vi "DilutionWalker.vi"() -> ()   [LabVIEW 2021]
uses:
  <userlib>/Nanonis Prog Interface V5/Nanonis Prog Interface.lvlib
panel:
  in  "Lockin offset (V)":dbl
  out "End":bool
  out "Pause":bool
  out "STM RX Temp":dbl=4.40353
  in  "STM RX\nTemperature Limit (K)":dbl=5.0
  out "Mix Chamber Temp":dbl=0.372436
  in  "Wait time (ms)":i32=1000
  in  "X Cap Upper limit (mV)":dbl=0.285
  in  "X Cap Lower limit (mV)":dbl=0.21
  in  "Mixing Chamber\nTemperature Limit (K)":dbl=0.4
  in  "?":bool
  in  "Number of Steps Increment":i32=400
  out "Z capacitance (pA)":cluster{"y":i32, sgl}[](graph)=[{"y"=0, -0.26452944}, {"y"=200, -0.27056125}, {"y"=400, -0.3170625}, {"y"=600, -0.30098757}, {"y"=800, -0.3354134}, {"y"=1000, -0.29213223}, {"y"=1200, -0.30642745}, {"y"=1400, -0.29814354}, {"y"=1600, -0.30608574}, {"y"=1800, -0.25005463}, {"y"=2000, -0.24961738}, {"y"=2200, -0.3531282}, {"y"=2400, -0.30892673}, {"y"=2600, -0.33144677}, {"y"=2800, -0.3248681}, {"y"=3000, -0.3031656}, {"y"=3200, -0.30311397}, {"y"=3400, -0.3312512}, {"y"=3600, -0.31709746}, {"y"=3800, -0.25381535}, {"y"=4000, -0.29973197}, {"y"=4200, -0.25194013}, {"y"=4400, -0.27562597}, {"y"=4600, -0.27429092}, {"y"=4800, -0.32395697}, {"y"=5000, -0.23664412}, {"y"=5200, -0.2965325}, {"y"=5400, -0.22288579}, {"y"=5600, -0.28061736}, {"y"=5800, -0.27647328}, {"y"=6000, -0.32065016}, {"y"=6200, -0.31318536}, {"y"=6400, -0.32285127}, {"y"=6600, -0.31599003}, {"y"=6800, -0.30435067}, {"y"=7000, -0.31278306}, {"y"=7200, -0.3015731}, {"y"=7400, -0.23340864}, {"y"=7600, -0.31077635}, {"y"=7800, -0.30132312}, {"y"=8000, -0.27798784}, {"y"=8200, -0.33925742}, {"y"=8400, -0.28044957}, {"y"=8600, -0.27736}, {"y"=8800, -0.26748103}, {"y"=9000, -0.26297227}, {"y"=9200, -0.35384896}, {"y"=9400, -0.28351077}, {"y"=9600, -0.27015728}, {"y"=9800, -0.2900495}, {"y"=10000, -0.30096906}, {"y"=10200, -0.34584683}, {"y"=10400, -0.33333805}, {"y"=10600, -0.25753516}, {"y"=10800, -0.32054728}, {"y"=11000, -0.33541495}, {"y"=11200, -0.30325446}, {"y"=11400, -0.24681602}, {"y"=11600, -0.28720984}, {"y"=11800, -0.32199413}, {"y"=12000, -0.34654015}, {"y"=12200, -0.25113922}, {"y"=12400, -0.31027225}, {"y"=12600, -0.2965383}, {"y"=12800, -0.314928}, {"y"=13000, -0.34754327}, {"y"=13200, -0.2174063}, {"y"=13400, -0.3269226}, {"y"=13600, -0.3417576}, {"y"=13800, -0.34317303}, {"y"=14000, -0.30799103}, {"y"=14200, -0.3409932}, {"y"=14400, -0.374583}, {"y"=14600, -0.3127186}, {"y"=14800, -0.36349568}, {"y"=15000, -0.32258537}, {"y"=15200, -0.35234475}, {"y"=15400, -0.26450554}, {"y"=15600, -0.31535837}, {"y"=15800, -0.29797876}, {"y"=16000, -0.37099135}, {"y"=16200, -0.3595007}, {"y"=16400, -0.3029738}, {"y"=16600, -0.3430387}, {"y"=16800, -0.32379654}, {"y"=17000, -0.2897029}, {"y"=17200, -0.35686213}, {"y"=17400, -0.32995725}, {"y"=17600, -0.3243773}, {"y"=17800, -0.27956468}, {"y"=18000, -0.33224046}, {"y"=18200, -0.26174507}, {"y"=18400, -0.2720899}, {"y"=18600, -0.31190276}, {"y"=18800, -0.365169}, {"y"=19000, -0.35901952}, {"y"=19200, -0.3133453}, {"y"=19400, -0.321272}, {"y"=19600, -0.3650524}, {"y"=19800, -0.3569558}, {"y"=20000, -0.3226467}, {"y"=20200, -0.3186869}, {"y"=20400, -0.27690017}, {"y"=20600, -0.29333174}, {"y"=20800, -0.3650037}, {"y"=21000, -0.34175736}, {"y"=21200, -0.30235806}, {"y"=21400, -0.30519643}, {"y"=21600, -0.33016568}, {"y"=21800, -0.268843}, {"y"=22000, -0.30949652}, {"y"=22200, -0.3402042}, {"y"=22400, -0.31630984}, {"y"=22600, -0.35675278}, {"y"=22800, -0.38607332}, {"y"=23000, -0.30069488}, {"y"=23200, -0.30392653}, {"y"=23400, -0.30562043}, {"y"=23600, -0.32636446}, {"y"=23800, -0.35105774}, {"y"=24000, -0.352251}, {"y"=24200, -0.27246413}, {"y"=24400, -0.32045224}, {"y"=24600, -0.30963522}, {"y"=24800, -0.3008064}, {"y"=25000, -0.2882819}, {"y"=25200, -0.24162695}, {"y"=25400, -0.3588808}, {"y"=25600, -0.37624997}, {"y"=25800, -0.33530983}, {"y"=26000, -0.32908398}, {"y"=26200, -0.36574924}, {"y"=26400, -0.36143667}, {"y"=26600, -0.31042248}, {"y"=26800, -0.28622916}, {"y"=27000, -0.32861832}, {"y"=27200, -0.35194245}, {"y"=27400, -0.2839697}, {"y"=27600, -0.3729146}, {"y"=27800, -0.35619572}, {"y"=28000, -0.31095412}, {"y"=28200, -0.32930008}, {"y"=28400, -0.3850868}, {"y"=28600, -0.3546264}, {"y"=28800, -0.29183277}, {"y"=29000, -0.25951427}, {"y"=29200, -0.34055057}, {"y"=29400, -0.30871165}, {"y"=29600, -0.33900478}, {"y"=29800, -0.26332897}, {"y"=30000, -0.34367266}, {"y"=30200, -0.3274469}, {"y"=30400, -0.3054115}, {"y"=30600, -0.27346995}, {"y"=30800, -0.3273148}, {"y"=31000, -0.30582932}, {"y"=31200, -0.27342635}, {"y"=31400, -0.3353544}, {"y"=31600, -0.3352716}, {"y"=31800, -0.31236312}, {"y"=32000, -0.29076076}, {"y"=32200, -0.30152094}, {"y"=32400, -0.35034788}, {"y"=32600, -0.265896}, {"y"=32800, -0.31590983}, {"y"=33000, -0.31764394}, {"y"=33200, -0.3159363}, {"y"=33400, -0.34009102}, {"y"=33600, -0.29582712}, {"y"=33800, -0.3217109}, {"y"=34000, -0.25372702}, {"y"=34200, -0.24392112}, {"y"=34400, -0.28812993}, {"y"=34600, -0.28951606}, {"y"=34800, -0.3079025}, {"y"=35000, -0.33620673}, {"y"=35200, -0.292474}, {"y"=35400, -0.3607892}, {"y"=35600, -0.27421385}, {"y"=35800, -0.3280191}, {"y"=36000, -0.302316}, {"y"=36200, -0.32416925}, {"y"=36400, -0.34789872}, {"y"=36600, -0.3196872}, {"y"=36800, -0.32483512}, {"y"=37000, -0.26164752}, {"y"=37200, -0.2820668}, {"y"=37400, -0.30672884}, {"y"=37600, -0.3690237}, {"y"=37800, -0.30537617}, {"y"=38000, -0.3308374}, {"y"=38200, -0.31725284}, {"y"=38400, -0.36457232}, {"y"=38600, -0.3042373}, {"y"=38800, -0.30165693}, {"y"=39000, -0.33604917}, {"y"=39200, -0.35489634}, {"y"=39400, -0.2743292}, {"y"=39600, -0.29021338}, {"y"=39800, -0.30953702}, {"y"=40000, -0.3207827}, {"y"=40200, -0.3375588}, {"y"=40400, -0.21972783}, {"y"=40600, -0.33964434}, {"y"=40800, -0.27738118}, {"y"=41000, -0.29640958}, {"y"=41200, -0.3743232}, {"y"=41400, -0.25270778}, {"y"=41600, -0.3212443}, {"y"=41800, -0.2828819}, {"y"=42000, -0.32858887}, {"y"=42200, -0.31920588}, {"y"=42400, -0.28080276}, {"y"=42600, -0.3156575}, {"y"=42800, -0.29654214}, {"y"=43000, -0.334953}, {"y"=43200, -0.33291087}, {"y"=43400, -0.33731157}, {"y"=43600, -0.29409498}, {"y"=43800, -0.29746836}, {"y"=44000, -0.31584385}, {"y"=44200, -0.39908078}, {"y"=44400, -0.28772417}, {"y"=44600, -0.28497294}, {"y"=44800, -0.28721952}, {"y"=45000, -0.31769314}, {"y"=45200, -0.25906157}, {"y"=45400, -0.3401025}, {"y"=45600, -0.2770137}, {"y"=45800, -0.30092195}, {"y"=46000, -0.30380133}, {"y"=46200, -0.33371064}, {"y"=46400, -0.3082187}, {"y"=46600, -0.36706933}, {"y"=46800, -0.28566322}, {"y"=47000, -0.30453646}, {"y"=47200, -0.2129875}, {"y"=47400, -0.35215983}, {"y"=47600, -0.30520058}, {"y"=47800, -0.38486058}, {"y"=48000, -0.30373412}, {"y"=48200, -0.3050348}, {"y"=48400, -0.25940648}, {"y"=48600, -0.3414501}, {"y"=48800, -0.29289445}, {"y"=49000, -0.3197257}, {"y"=49200, -0.28932348}, {"y"=49400, -0.26191166}, {"y"=49600, -0.19608292}, {"y"=49800, -0.3571897}, {"y"=50000, -0.32131934}, {"y"=50200, -0.30441958}, {"y"=50400, -0.32406878}, {"y"=50600, -0.34500462}, {"y"=50800, -0.34577286}, {"y"=51000, -0.27084503}, {"y"=51200, 0.008703331}, {"y"=51400, -0.5370679}, {"y"=51600, -0.28328782}, {"y"=51800, -0.31837463}, {"y"=52000, -0.28617984}, {"y"=52200, -0.2819138}, {"y"=52400, -0.31492892}, {"y"=52600, -0.28859508}, {"y"=52800, -0.30150834}, {"y"=53000, -0.26601008}, {"y"=53200, -0.28601724}, {"y"=53400, -0.2551962}, {"y"=53600, -0.30998704}, {"y"=53800, -0.29331136}, {"y"=54000, -0.24365473}, {"y"=54200, -0.2894879}]
  out "X capacitance (mV)":cluster{"y":i32, dbl}[](graph)=[{"y"=0, 0.21357266902923586}, {"y"=200, 0.2147012710571289}, {"y"=400, 0.21581780910491943}, {"y"=600, 0.21690545082092286}, {"y"=800, 0.2179858684539795}, {"y"=1000, 0.21903662681579592}, {"y"=1200, 0.22008056640625}, {"y"=1400, 0.22109785079956054}, {"y"=1600, 0.22207918167114257}, {"y"=1800, 0.2231245517730713}, {"y"=2000, 0.2240769386291504}, {"y"=2200, 0.22501637935638427}, {"y"=2400, 0.22596323490142822}, {"y"=2600, 0.2268744945526123}, {"y"=2800, 0.22776687145233154}, {"y"=3000, 0.22866487503051758}, {"y"=3200, 0.229524302482605}, {"y"=3400, 0.23036799430847169}, {"y"=3600, 0.2312250852584839}, {"y"=3800, 0.23205804824829102}, {"y"=4000, 0.23286981582641603}, {"y"=4200, 0.23366889953613282}, {"y"=4400, 0.234482216835022}, {"y"=4600, 0.23526401519775392}, {"y"=4800, 0.23600375652313232}, {"y"=5000, 0.23675258159637452}, {"y"=5200, 0.23748691082000734}, {"y"=5400, 0.2381901264190674}, {"y"=5600, 0.2389019250869751}, {"y"=5800, 0.23960814476013184}, {"y"=6000, 0.24029965400695802}, {"y"=6200, 0.24096741676330566}, {"y"=6400, 0.24164459705352784}, {"y"=6600, 0.2423039197921753}, {"y"=6800, 0.24296264648437502}, {"y"=7000, 0.24360923767089845}, {"y"=7200, 0.2442251205444336}, {"y"=7400, 0.24485447406768798}, {"y"=7600, 0.2454981565475464}, {"y"=7800, 0.24609751701354982}, {"y"=8000, 0.2466892719268799}, {"y"=8200, 0.24729080200195314}, {"y"=8400, 0.2478795051574707}, {"y"=8600, 0.24845747947692873}, {"y"=8800, 0.24902808666229248}, {"y"=9000, 0.24959423542022705}, {"y"=9200, 0.2501417398452759}, {"y"=9400, 0.2507206678390503}, {"y"=9600, 0.25126259326934813}, {"y"=9800, 0.25181381702423095}, {"y"=10000, 0.2523436784744263}, {"y"=10200, 0.25286843776702883}, {"y"=10400, 0.2534111738204956}, {"y"=10600, 0.25392258167266846}, {"y"=10800, 0.2544567346572876}, {"y"=11000, 0.254944896697998}, {"y"=11200, 0.2554523706436157}, {"y"=11400, 0.2559502363204956}, {"y"=11600, 0.2564888000488281}, {"y"=11800, 0.2569794416427612}, {"y"=12000, 0.2574486017227173}, {"y"=12200, 0.25792760848999025}, {"y"=12400, 0.2583930253982544}, {"y"=12600, 0.2588639259338379}, {"y"=12800, 0.25932180881500244}, {"y"=13000, 0.25977411270141604}, {"y"=13200, 0.26023385524749754}, {"y"=13400, 0.2606536626815796}, {"y"=13600, 0.26108036041259763}, {"y"=13800, 0.2615255832672119}, {"y"=14000, 0.26193556785583494}, {"y"=14200, 0.2623560428619385}, {"y"=14400, 0.26276822090148927}, {"y"=14600, 0.2631711483001709}, {"y"=14800, 0.2635857343673706}, {"y"=15000, 0.26398282051086425}, {"y"=15200, 0.26438772678375244}, {"y"=15400, 0.26477880477905275}, {"y"=15600, 0.2651677131652832}, {"y"=15800, 0.26553940773010254}, {"y"=16000, 0.2659076929092407}, {"y"=16200, 0.2662929058074951}, {"y"=16400, 0.26666946411132814}, {"y"=16600, 0.2670249938964844}, {"y"=16800, 0.2674261569976807}, {"y"=17000, 0.2678008794784546}, {"y"=17200, 0.26815156936645507}, {"y"=17400, 0.26851491928100585}, {"y"=17600, 0.26885788440704345}, {"y"=17800, 0.2691839694976807}, {"y"=18000, 0.26951904296875}, {"y"=18200, 0.2698603868484497}, {"y"=18400, 0.27021329402923583}, {"y"=18600, 0.2705530643463135}, {"y"=18800, 0.2708828210830689}, {"y"=19000, 0.2712192296981812}, {"y"=19200, 0.2715223789215088}, {"y"=19400, 0.2718502998352051}, {"y"=19600, 0.2721735954284668}, {"y"=19800, 0.2724856615066528}, {"y"=20000, 0.27282190322875977}, {"y"=20200, 0.2731217622756958}, {"y"=20400, 0.27344110012054446}, {"y"=20600, 0.27374932765960697}, {"y"=20800, 0.27404532432556156}, {"y"=21000, 0.27433764934539795}, {"y"=21200, 0.2746425151824951}, {"y"=21400, 0.2749338150024414}, {"y"=21600, 0.2752199411392212}, {"y"=21800, 0.27551238536834716}, {"y"=22000, 0.2758016586303711}, {"y"=22200, 0.2760864019393921}, {"y"=22400, 0.27636544704437255}, {"y"=22600, 0.27662317752838134}, {"y"=22800, 0.2768929719924927}, {"y"=23000, 0.2771783828735352}, {"y"=23200, 0.2774518013000488}, {"y"=23400, 0.27770495414733887}, {"y"=23600, 0.27798678874969485}, {"y"=23800, 0.27826545238494876}, {"y"=24000, 0.27853381633758545}, {"y"=24200, 0.27880263328552246}, {"y"=24400, 0.27903494834899906}, {"y"=24600, 0.2792867183685303}, {"y"=24800, 0.27953026294708255}, {"y"=25000, 0.27976553440093993}, {"y"=25200, 0.27997915744781493}, {"y"=25400, 0.2802250385284424}, {"y"=25600, 0.2804482221603394}, {"y"=25800, 0.28068132400512696}, {"y"=26000, 0.28090481758117675}, {"y"=26200, 0.2811241865158081}, {"y"=26400, 0.28135080337524415}, {"y"=26600, 0.28156116008758547}, {"y"=26800, 0.2817727088928223}, {"y"=27000, 0.28198957443237305}, {"y"=27200, 0.2822116374969483}, {"y"=27400, 0.28240485191345216}, {"y"=27600, 0.28261585235595704}, {"y"=27800, 0.2828121900558472}, {"y"=28000, 0.28301324844360354}, {"y"=28200, 0.2831972360610962}, {"y"=28400, 0.28341150283813477}, {"y"=28600, 0.2835517644882202}, {"y"=28800, 0.28375835418701173}, {"y"=29000, 0.28395938873291016}, {"y"=29200, 0.2841550588607788}, {"y"=29400, 0.28433682918548586}, {"y"=29600, 0.284511923789978}, {"y"=29800, 0.28469271659851075}, {"y"=30000, 0.2848948955535889}, {"y"=30200, 0.28506882190704347}, {"y"=30400, 0.2852374076843262}, {"y"=30600, 0.2854273080825806}, {"y"=30800, 0.2855900764465332}, {"y"=31000, 0.28576691150665284}, {"y"=31200, 0.2859371662139893}, {"y"=31400, 0.2861051082611084}, {"y"=31600, 0.2862806081771851}, {"y"=31800, 0.2864513874053955}, {"y"=32000, 0.28663358688354496}, {"y"=32200, 0.2867846727371216}, {"y"=32400, 0.2869489431381226}, {"y"=32600, 0.2871151685714722}, {"y"=32800, 0.2872730016708374}, {"y"=33000, 0.28744561672210694}, {"y"=33200, 0.2875957250595093}, {"y"=33400, 0.2877490758895874}, {"y"=33600, 0.28789725303649905}, {"y"=33800, 0.2880505323410034}, {"y"=34000, 0.2882134437561035}, {"y"=34200, 0.2883355140686035}, {"y"=34400, 0.2884969234466553}, {"y"=34600, 0.28863437175750734}, {"y"=34800, 0.28878488540649416}, {"y"=35000, 0.2889194250106812}, {"y"=35200, 0.2890756130218506}, {"y"=35400, 0.2892141819000244}, {"y"=35600, 0.2894058465957642}, {"y"=35800, 0.28953988552093507}, {"y"=36000, 0.28968157768249514}, {"y"=36200, 0.2898248672485352}, {"y"=36400, 0.28995480537414553}, {"y"=36600, 0.2900970697402954}, {"y"=36800, 0.29024991989135746}, {"y"=37000, 0.2903444528579712}, {"y"=37200, 0.29047365188598634}, {"y"=37400, 0.2906097650527954}, {"y"=37600, 0.29073963165283206}, {"y"=37800, 0.29086334705352784}, {"y"=38000, 0.29100320339202884}, {"y"=38200, 0.2911355495452881}, {"y"=38400, 0.2912521123886109}, {"y"=38600, 0.29138960838317873}, {"y"=38800, 0.29152185916900636}, {"y"=39000, 0.29163422584533694}, {"y"=39200, 0.2917720556259155}, {"y"=39400, 0.2919000625610352}, {"y"=39600, 0.29201946258544925}, {"y"=39800, 0.2921566724777222}, {"y"=40000, 0.29228351116180423}, {"y"=40200, 0.2924021005630493}, {"y"=40400, 0.29252257347106936}, {"y"=40600, 0.29265565872192384}, {"y"=40800, 0.2927766084671021}, {"y"=41000, 0.2928893804550171}, {"y"=41200, 0.29299316406250003}, {"y"=41400, 0.293117880821228}, {"y"=41600, 0.29324495792388916}, {"y"=41800, 0.29335086345672606}, {"y"=42000, 0.2934612512588501}, {"y"=42200, 0.2935697317123413}, {"y"=42400, 0.29368646144866944}, {"y"=42600, 0.29380550384521487}, {"y"=42800, 0.293912148475647}, {"y"=43000, 0.2940265417098999}, {"y"=43200, 0.2941251277923584}, {"y"=43400, 0.2942491054534912}, {"y"=43600, 0.29435300827026367}, {"y"=43800, 0.29446349143981937}, {"y"=44000, 0.29457106590271}, {"y"=44200, 0.2946788311004639}, {"y"=44400, 0.2947965145111084}, {"y"=44600, 0.2949222087860108}, {"y"=44800, 0.29503176212310794}, {"y"=45000, 0.2951323747634888}, {"y"=45200, 0.29524805545806887}, {"y"=45400, 0.2953538417816162}, {"y"=45600, 0.29539966583251953}, {"y"=45800, 0.2955051898956299}, {"y"=46000, 0.29560346603393556}, {"y"=46200, 0.2957145929336548}, {"y"=46400, 0.29580819606781006}, {"y"=46600, 0.29591619968414307}, {"y"=46800, 0.2960115909576416}, {"y"=47000, 0.29612088203430176}, {"y"=47200, 0.2962247610092163}, {"y"=47400, 0.29632201194763186}, {"y"=47600, 0.2964148044586182}, {"y"=47800, 0.296518611907959}, {"y"=48000, 0.29661657810211184}, {"y"=48200, 0.2967301368713379}, {"y"=48400, 0.29681997299194335}, {"y"=48600, 0.29692456722259525}, {"y"=48800, 0.2970076322555542}, {"y"=49000, 0.2971181392669678}, {"y"=49200, 0.29723029136657714}, {"y"=49400, 0.2972947359085083}, {"y"=49600, 0.2974052667617798}, {"y"=49800, 0.29750559329986576}, {"y"=50000, 0.2976086616516113}, {"y"=50200, 0.29770348072052005}, {"y"=50400, 0.2977898597717285}, {"y"=50600, 0.297877836227417}, {"y"=50800, 0.297983193397522}, {"y"=51000, 0.29804625511169436}, {"y"=51200, 0.29815452098846434}, {"y"=51400, 0.29822735786437987}, {"y"=51600, 0.2983759164810181}, {"y"=51800, 0.29846811294555664}, {"y"=52000, 0.2985581159591675}, {"y"=52200, 0.2986560583114624}, {"y"=52400, 0.2987450838088989}, {"y"=52600, 0.298833703994751}, {"y"=52800, 0.29891486167907716}, {"y"=53000, 0.2989931344985962}, {"y"=53200, 0.2990796804428101}, {"y"=53400, 0.29915268421173097}, {"y"=53600, 0.2992403984069824}, {"y"=53800, 0.29933180809021}, {"y"=54000, 0.29941155910491946}, {"y"=54200, 0.2994891405105591}]
  in  "Lockin sensitivity (V)":dbl=0.001
  out "X capacitance (mV)":sgl=0.29948914
  out "Current (pA)":sgl=0.15895681
  out "Z capacitance (pA)":sgl=-0.2894879
  # "+X"
  # "-X"
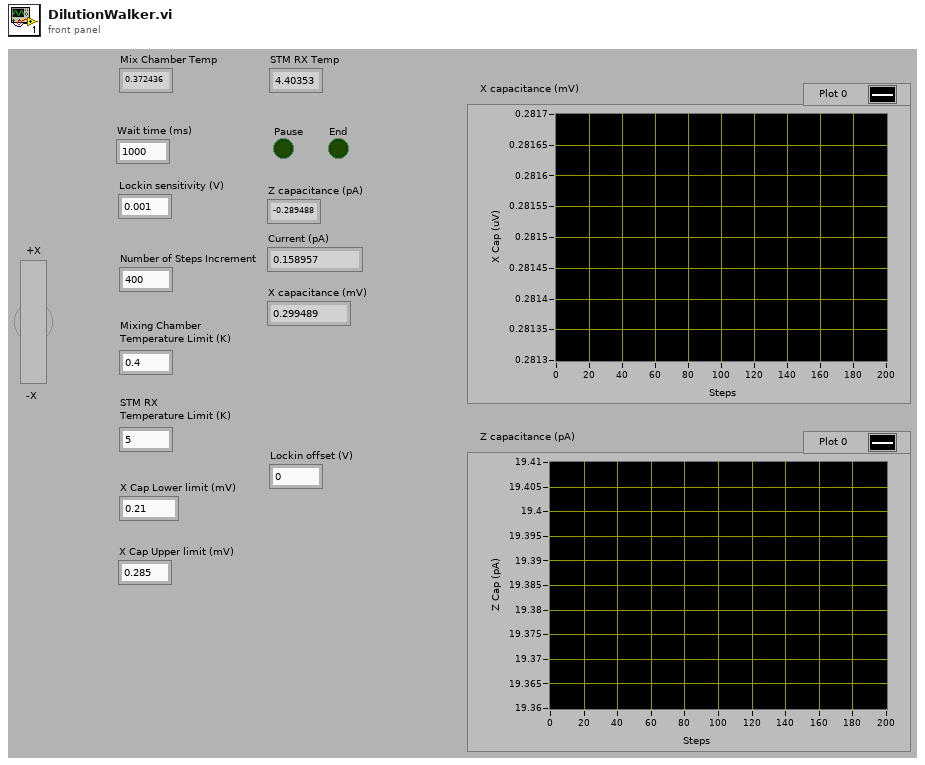
[diagram p1: front panel]
types:
  T1 = enum16{"Set Heater Voltage", "Read Heater Voltage", "Read Heater Current", "Read 1K Pot Temperature", "Read IVC Sorb Temperature", "Read Needle Valve Temperature", "Read Still Pressure", "Read Mixing Chamber Temperature", "Read STM RX Temperature", "Read STM CX Temperature", "Unstall Triton Loop", "Triton Stop", "Triton Stall Status"}
  T2 = enum8{"Group 1", "Group 2", "Group 3", "Group 4", "Group 5", "Group 6"}
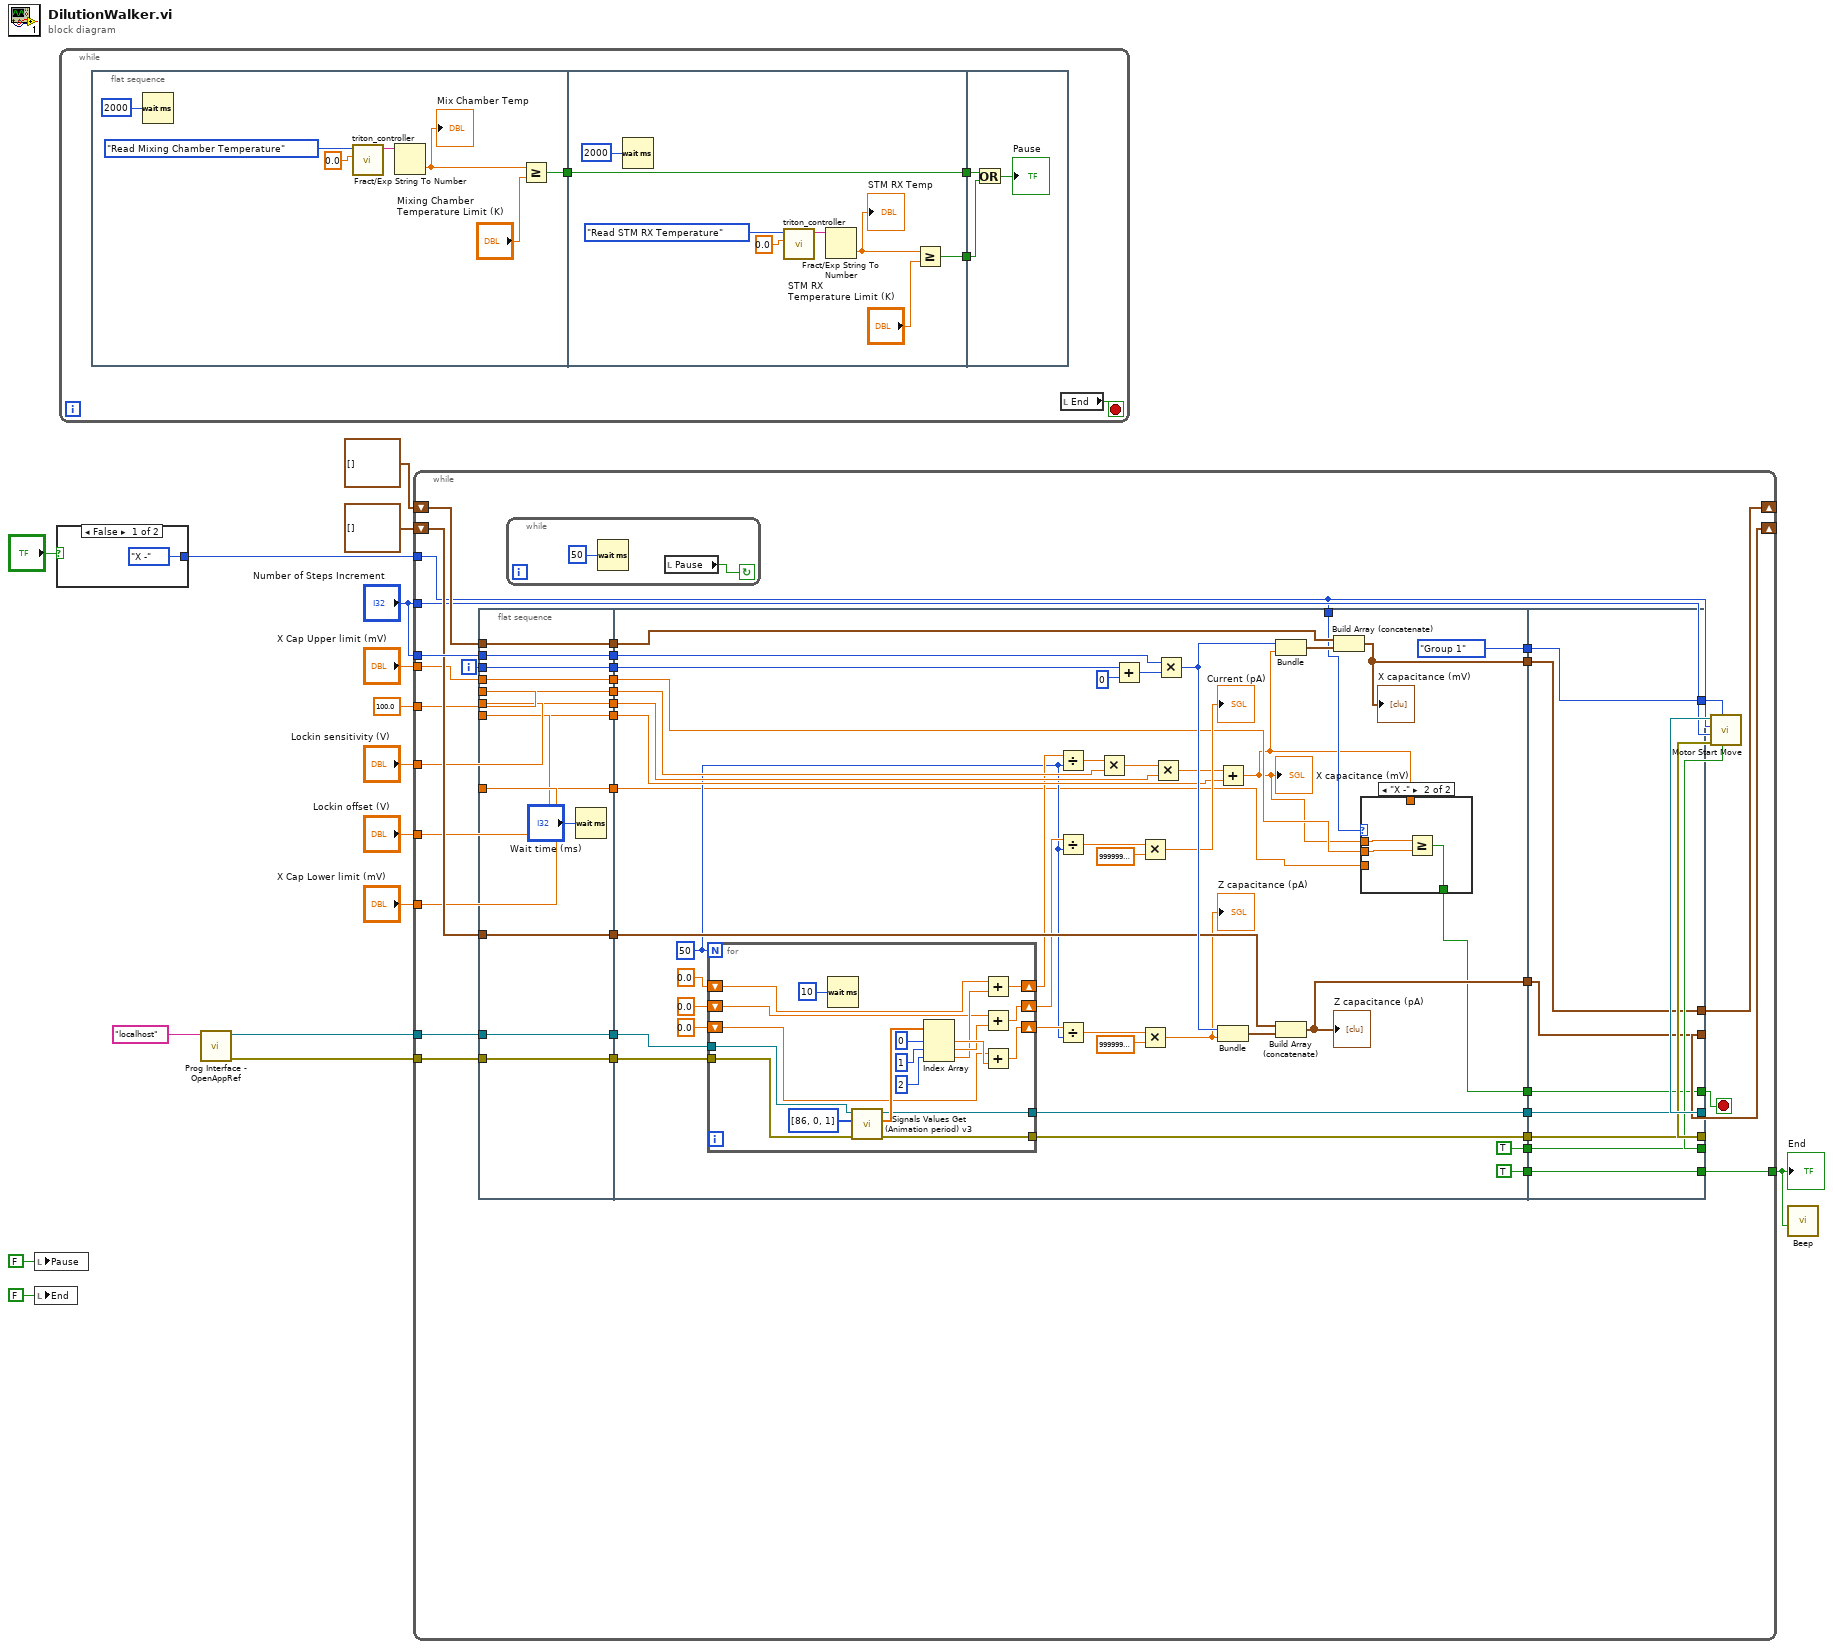
[diagram p0: block diagram]
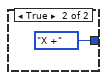
[diagram p2: hidden frame]
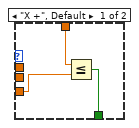
[diagram p3: hidden frame]
diagram:
  n1 = local write "Pause"(FALSE ("Pause")) -> ()
  n2 = local write "End"(FALSE ("End")) -> ()
  n3 = case shown="False" "?" {
    tunnel: [enum16{"X +", "X -", "Y +", "Y -", "Z +", "Z -"}."X -" ("Direction") enum16{"X +", "X -", "Y +", "Y -", "Z +", "Z -"}."X +" ("Direction")] -> w14
    frame False {
    }
    frame True {
    }
  }
  n4 = while {
    stop <- w19 stop-if-true
    n5 = flat-sequence {
      tunnel: [w23] -> w20
      tunnel: [w31] -> w22
      tunnel: [w30] -> w21
      tunnel: w20 -> [w30]
      tunnel: w22 -> [w40]
      tunnel: w21 -> [w39]
      frame #0 {
        n6 = Wait (ms)(milliseconds to wait=u32 2000) -> ()  [unwired: 1 out]
        n7 = call "triton_controller.vi"("Numerical Argument"=0.0, "Command"=T1."Read Mixing Chamber Temperature") -> ("Response"=w26:string)  [unwired: 9 in]
        n8 = Fract/Exp String To Number(string=w26) -> (number=w25:dbl)  [unwired: 3 in, 1 out]
        "Mix Chamber Temp" <- w25
        n9 = Greater Or Equal?(x=w25, y="Mixing Chamber\nTemperature Limit (K)") -> (x >= y?=w23:bool)
      }
      frame #1 {
        n10 = Wait (ms)(milliseconds to wait=u32 2000) -> ()  [unwired: 1 out]
        n11 = call "triton_controller.vi"("Numerical Argument"=0.0, "Command"=T1."Read STM RX Temperature") -> ("Response"=w34:string)  [unwired: 9 in]
        n12 = Fract/Exp String To Number(string=w34) -> (number=w32:dbl)  [unwired: 3 in, 1 out]
        "STM RX Temp" <- w32
        n13 = Greater Or Equal?(x=w32, y="STM RX\nTemperature Limit (K)") -> (x >= y?=w31:bool)
      }
      frame #2 {
        n14 = Or(x=w39, y=w40) -> (x .or. y?=→"Pause":bool)
      }
    }
    n15 = local read "End"() -> (w19:bool)
  }
  n16 = call <userlib>:"Prog Interface - OpenAppRef.vi"("Machine name (local machine IP)"="localhost" ("machine name (localhost)")) -> ("Error out"=w1:errorcluster, "Application reference"=w2:refnum<vi>)  [unwired: 5 in]
  n17 = while {
    tunnel: w1 -> [w80]
    tunnel: w2 -> [w79]
    tunnel: "Lockin sensitivity (V)" -> [w65]
    tunnel: "Number of Steps Increment" -> [w78]
    shift-right: [w68] -> _
    shift-left: cluster{i32, sgl}[] [] -> [w77]
    shift-right: [w69] -> _
    shift-left: cluster{i32, sgl}[] [] -> [w76]
    tunnel: w14 -> [w43]
    tunnel: "Number of Steps Increment" -> [w72]
    tunnel: [w70] -> w12
    tunnel: 100.0 ("y") -> [w67]
    tunnel: "X Cap Upper limit (mV)" -> [w64]
    tunnel: "X Cap Lower limit (mV)" -> [w63]
    tunnel: "Lockin offset (V)" -> [w62]
    i -> [w66]
    stop <- w42 stop-if-true
    n18 = flat-sequence {
      tunnel: w62 -> [w82]
      tunnel: w63 -> [w83]
      tunnel: w64 -> [w84]
      tunnel: w65 -> [w85]
      tunnel: w66 -> [w86]
      tunnel: w67 -> [w87]
      tunnel: w76 -> [w88]
      tunnel: w77 -> [w89]
      tunnel: w78 -> [w90]
      tunnel: w79 -> [w91]
      tunnel: w80 -> [w92]
      tunnel: [w92] -> w54
      tunnel: [w91] -> w53
      tunnel: [w90] -> w52
      tunnel: [w89] -> w51
      tunnel: [w88] -> w50
      tunnel: [w87] -> w49
      tunnel: [w86] -> w48
      tunnel: [w85] -> w47
      tunnel: [w84] -> w46
      tunnel: [w83] -> w45
      tunnel: [w82] -> w44
      tunnel: [w122] -> w61
      tunnel: [w121] -> w60
      tunnel: [TRUE ("Wait until finished? (F)")] -> w59
      tunnel: [T2."Group 1" ("Group")] -> w58
      tunnel: [TRUE] -> w57
      tunnel: [w117] -> w56
      tunnel: [w116] -> w55
      tunnel: w54 -> [w134]
      tunnel: w53 -> [w133]
      tunnel: w52 -> [w128]
      tunnel: w51 -> [w126]
      tunnel: w50 -> [w123]
      tunnel: w49 -> [w115]
      tunnel: w48 -> [w112]
      tunnel: w47 -> [w111]
      tunnel: w46 -> [w96]
      tunnel: w45 -> [w94]
      tunnel: w44 -> [w108]
      tunnel: w43 -> [w97]
      tunnel: [w93] -> w41
      tunnel: [w161] -> w68
      tunnel: [w162] -> w69
      tunnel: [w163] -> w70
      tunnel: [w164] -> w71
      tunnel: [w165] -> w73
      tunnel: [w166] -> w74
      tunnel: [w167] -> w75
      tunnel: w61 -> [w167]
      tunnel: w60 -> [w166]
      tunnel: w59 -> [w165]
      tunnel: w58 -> [w164]
      tunnel: w57 -> [w163]
      tunnel: w56 -> [w162]
      tunnel: w55 -> [w161]
      tunnel: [w160] -> w42
      tunnel: w41 -> [w160]
      frame #0 {
        n19 = Wait (ms)(milliseconds to wait="Wait time (ms)") -> ()  [unwired: 1 out]
      }
      frame #1 {
        w98 = 50
        n20 = for {
          N: w98 -> [_]
          tunnel: w134 -> [w159]
          tunnel: w133 -> [w155]
          tunnel: [w152] -> w122
          tunnel: [w151] -> w121
          shift-right: [w148] -> w103
          shift-left: sgl 0.0 -> [w143]
          shift-right: [w147] -> w99
          shift-left: sgl 0.0 -> [w142]
          shift-right: [w144] -> w101
          shift-left: sgl 0.0 -> [w141]
          n21 = Wait (ms)(milliseconds to wait=u32 10) -> ()  [unwired: 1 out]
          n22 = call <userlib>:"Signals Values Get (Animation period) v3.vi"("error in (no error)"=w159, "Signals indexes (0-127)"=i8[] [86, 0, 1], "Application ref in"=w155) -> ("error out"=w151:errorcluster, "Signals Values"=w157:sgl[], "Application ref out"=w152:refnum<vi>)  [unwired: 5 in]
          n23 = Index Array(array=w157, index #1=0 ("index"), index #2=1 ("index"), index #3=2 ("index")) -> (element #1=w149:sgl, element #2=w146:sgl, element #3=w145:sgl)
          n24 = Add(x=w141, y=w145) -> (x+y=w144:sgl)
          n25 = Add(x=w142, y=w146) -> (x+y=w147:sgl)
          n26 = Add(x=w143, y=w149) -> (x+y=w148:sgl)
        }
        n27 = Divide(x=w101, y=w98) -> (x/y=w102:sgl)
        n28 = Divide(x=w99, y=w98) -> (x/y=w100:sgl)
        n29 = Divide(x=w103, y=w98) -> (x/y=w104:sgl)
        n30 = Multiply(x=w102, y=w115) -> (x*y=w110:dbl)
        n31 = Add(x=w112, y=u16 0) -> (x+y=w129:i32)
        n32 = Multiply(x=w100, y=sgl 1000000000000.0) -> (x*y=→"Current (pA)":sgl)
        n33 = Multiply(x=w104, y=sgl 1000000000000.0) -> (x*y=w113:sgl)
        "Z capacitance (pA)" <- w113
        n34 = Multiply(x=w110, y=w111) -> (x*y=w109:dbl)
        n35 = Multiply(x=w128, y=w129) -> (x*y=w125:i32)
        n36 = Add(x=w109, y=w108) -> (x+y=w95:dbl)
        "X capacitance (mV)" <- w95
        n37 = Bundle(w125, w113) -> (w124:cluster{i32, sgl})  [unwired: 1 in]
        n38 = Bundle(w125, w95) -> (w127:cluster{i32, dbl})  [unwired: 1 in]
        n39 = Build Array (concatenate)(w123, w124) -> (w117:cluster{i32, sgl}[])
        "Z capacitance (pA)" <- w117
        n40 = Build Array (concatenate)(w126, w127) -> (w116:cluster{i32, dbl}[])
        "X capacitance (mV)" <- w116
        n41 = case shown="\"X -\"" w97 {
          tunnel: w95 -> [_ w140]
          tunnel: w96 -> [_ w139]
          tunnel: w95 -> [w137 _]
          tunnel: w94 -> [w136 _]
          tunnel: [w135 w138] -> w93
          frame "X +", Default {
            n42 = Less Or Equal?(x=w137, y=w136) -> (x <= y?=w135:bool)
          }
          frame "X -" {
            n43 = Greater Or Equal?(x=w140, y=w139) -> (x >= y?=w138:bool)
          }
        }
      }
      frame #2 {
      }
    }
    n44 = while {
      stop <- w169 continue-if-true
      n45 = Wait (ms)(milliseconds to wait=u32 50) -> ()  [unwired: 1 out]
      n46 = local read "Pause"() -> (w169:bool)
    }
    n47 = call <userlib>:"Motor Start Move.vi"("Wait until finished? (F)"=w73, "Group"=w71, "Error in (no error)"=w74, "Number of steps"=w72, "Direction"=w43, "Application ref in"=w75) -> ()  [unwired: 3 in, 2 out]
  }
  "End" <- w12
  n48 = call <vilib>:"Beep.vi"("use system alert? (T)"=w12) -> ()  [unwired: 11 in]
